vi "Sequence Settings Number to Cluster.vi"(1 "Sequence Settings":i32) -> (0 "Settings":T1)   [LabVIEW 2011]
uses:
  Sequence Settings.ctl
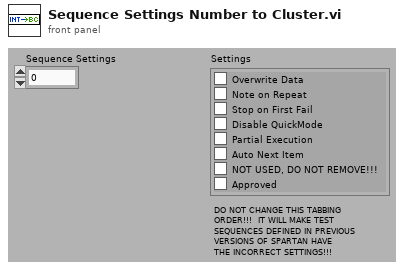
[diagram p1: front panel]
types:
  T1 = typedef "Sequence Settings.ctl" = cluster{"Overwrite Data":bool, "Note on Repeat":bool, "Stop on First Fail":bool, "Disable QuickMode":bool, "Partial Execution":bool, "Auto Next Item":bool, "NOT USED, DO NOT REMOVE!!!":bool, "Approved":bool}
  T2 = cluster{"Boolean array[0]":bool, "Boolean array[1]":bool, "Boolean array[2]":bool, "Boolean array[3]":bool, "Boolean array[4]":bool, "Boolean array[5]":bool, "Boolean array[6]":bool, "Boolean array[7]":bool}
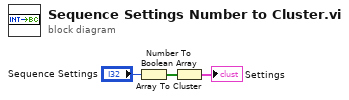
[diagram p0: block diagram]
diagram:
  n1 = Number To Boolean Array(number="Sequence Settings") -> (Boolean array=w1:bool[])
  n2 = Array To Cluster(array=w1) -> (cluster=→"Settings":T2)
